vi "FrontPenelControlRefFGV.vi"(7 "Action":enum16{"Read", "Write"}(ring), 10 "Write":T1) -> (2 "Read":T1)   [LabVIEW 2019, in "SME_Data_Acquisition.lvlib"]
uses:
  SME_Data_Acquisition.lvlib
  FrontPanelCtrlRef.ctl
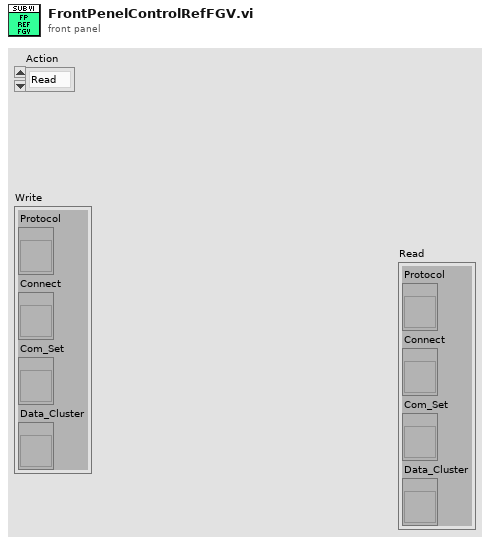
[diagram p1: front panel]
types:
  T1 = typedef "SME_Data_Acquisition.lvlib/FrontPanelCtrlRef.ctl" = cluster{"Protocol":refnum<vi>, "Connect":refnum<vi>, "Com_Set":refnum<vi>, "Data_Cluster":refnum<vi>}
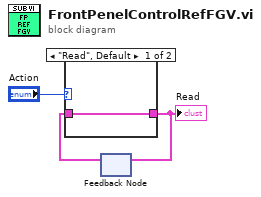
[diagram p0: block diagram]
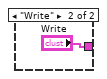
[diagram p2: hidden frame]
diagram:
  n1 = feedback #1() -> (w1:T1)  [unwired: 1 in]
  n2 = case shown="\"Read\", Default" "Action" {
    tunnel: [w4 "Write"] -> w2
    tunnel: w1 -> [w4 _]
    frame "Read", Default {
    }
    frame "Write" {
    }
  }
  "Read" <- w2
  n3 = feedback-in #1(w2) -> ()
